vi "GetMessage.vi"(7 "Action":enum16{"Blank", "Menu"}(ring)=enum."Menu", 8 "Error in":errorcluster, 11 "Message Type":string) -> (0 "Error Out":errorcluster, 1 "Right Menu":cluster{"R1":string, "R2":string, "R3":string}, 2 "Left menu":cluster{"L1":string, "L2":string, "L3":string}, 3 "Get Message":string)   [LabVIEW 2017]
doc: "This VI shows the menu messages and the Main ATM message as per the selection."
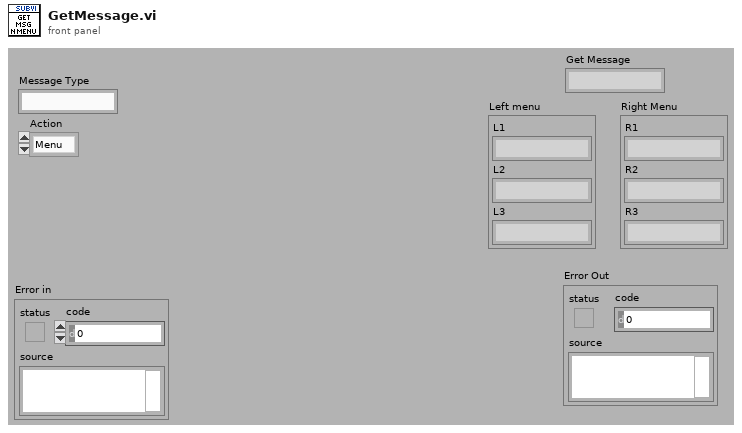
[diagram p1: front panel]
types:
  T1 = cluster{"Array[0]":string, "Array[1]":string, "Array[2]":string}
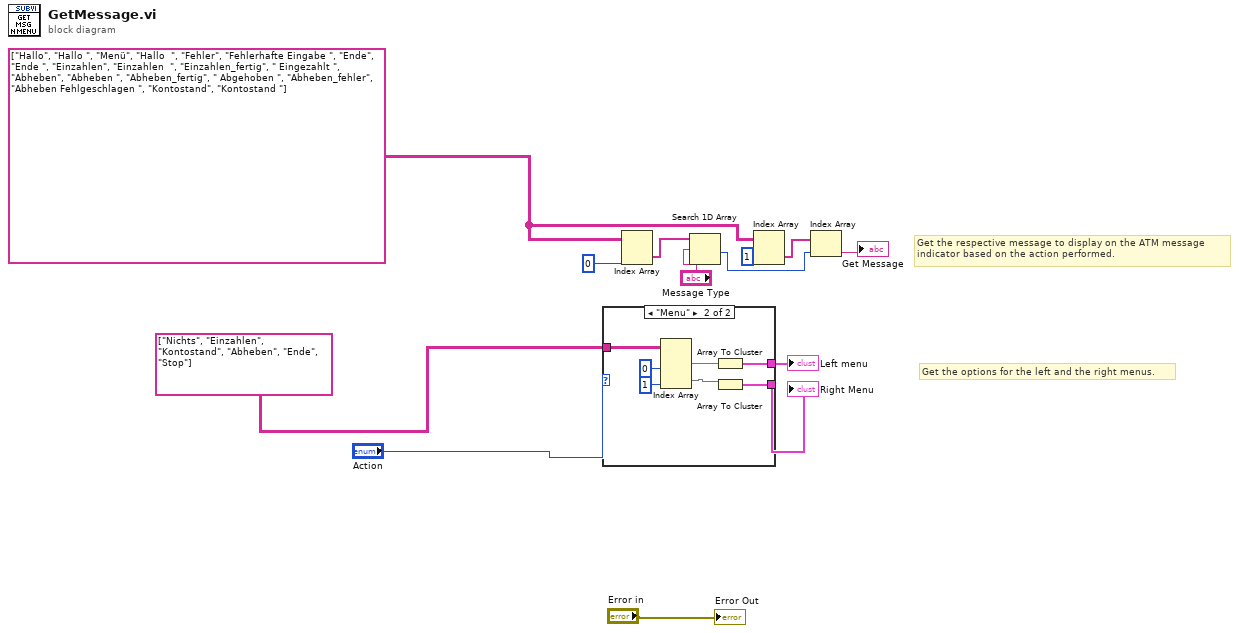
[diagram p0: block diagram]
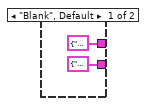
[diagram p2: hidden frame]
diagram:
  w1 = string[][] [["Hallo", "Hallo "], ["Menü", "Hallo  "], ["Fehler", "Fehlerhafte Eingabe "], ["Ende", "Ende "], ["Einzahlen", "Einzahlen  "], ["Einzahlen_fertig", " Eingezahlt "], ["Abheben", "Abheben "], ["Abheben_fertig", " Abgehoben "], ["Abheben_fehler", "Abheben Fehlgeschlagen "], ["Kontostand", "Kontostand "]] ("Array")
  # "Get the options for the left and the right menus."
  # "Get the respective message to display on the ATM message\nindicator based on the action performed."
  n1 = case shown="\"Menu\"" "Action" {
    tunnel: string[][] [["Nichts", "Einzahlen"], ["Kontostand", "Abheben"], ["Ende", "Stop"]] ("Array") -> [_ w22]
    tunnel: [T1 {"Array[0]"="", "Array[1]"="", "Array[2]"=""} ("Array") w17] -> w4
    tunnel: [T1 {"Array[0]"="", "Array[1]"="", "Array[2]"=""} ("Array") w16] -> w3
    frame "Blank", Default {
    }
    frame "Menu" {
      n2 = Index Array(array=w22, index (col) #1=0 ("disabled index (col)"), index (col) #2=1 ("index (col)")) -> (element #1=w21:string[], element #2=w20:string[])  [unwired: 2 in]
      n3 = Array To Cluster(array=w21) -> (cluster=w17:T1)
      n4 = Array To Cluster(array=w20) -> (cluster=w16:T1)
    }
  }
  "Left menu" <- w4
  "Right Menu" <- w3
  n5 = Index Array(array=w1, index (col)=0 ("disabled index (col)")) -> (element=w12:string[])  [unwired: 1 in]
  n6 = Search 1D Array(1D array=w12, element="Message Type") -> (index of element=w8:i32)  [unwired: 1 in]
  n7 = Index Array(array=w1, index (col)=1 ("disabled index (col)")) -> (element=w9:string[])  [unwired: 1 in]
  n8 = Index Array(array=w9, index=w8) -> (element=→"Get Message":string)
  "Error Out" <- "Error in"
